vi "mediaIntesecaoBlue.vi"(11 "Array":T4[](array[typedef]) {"robots_blue"."height" format="%+4.3f"; "robots_blue"."pixel_y" format="%+4.3f"; "robots_blue"."pixel_x" format="%+4.3f"; "robots_blue"."orientation" format="%+4.3f"; "robots_blue"."y" format="%+4.3f"; "robots_blue"."confidence" format="%4.3f"; "robots_blue"."x" format="%+4.3f"; "robots_yellow"."height" format="%+4.3f"; "robots_yellow"."pixel_y" format="%+4.3f"; "robots_yellow"."pixel_x" format="%+4.3f"; "robots_yellow"."orientation" format="%+4.3f"; "robots_yellow"."y" format="%+4.3f"; "robots_yellow"."confidence" format="%4.3f"; "robots_yellow"."x" format="%+4.3f"}) -> (3 "Array 2":T1[](array[typedef]) {"height" format="%+4.3f"; "pixel_y" format="%+4.3f"; "pixel_x" format="%+4.3f"; "orientation" format="%+4.3f"; "y" format="%+4.3f"; "confidence" format="%4.3f"; "x" format="%+4.3f"})   [LabVIEW 2018]
uses:
  SSL Detection Frame.ctl
  SSL Detection Robot.ctl
  <vilib>/Analysis/Matrix/Datatypes/RealMatrix.ctl
  SSL Detection Ball.ctl
  <vilib>/Analysis/Matrix/NI_Matrix.lvlib
panel:
  in  "Field Size 2":T3
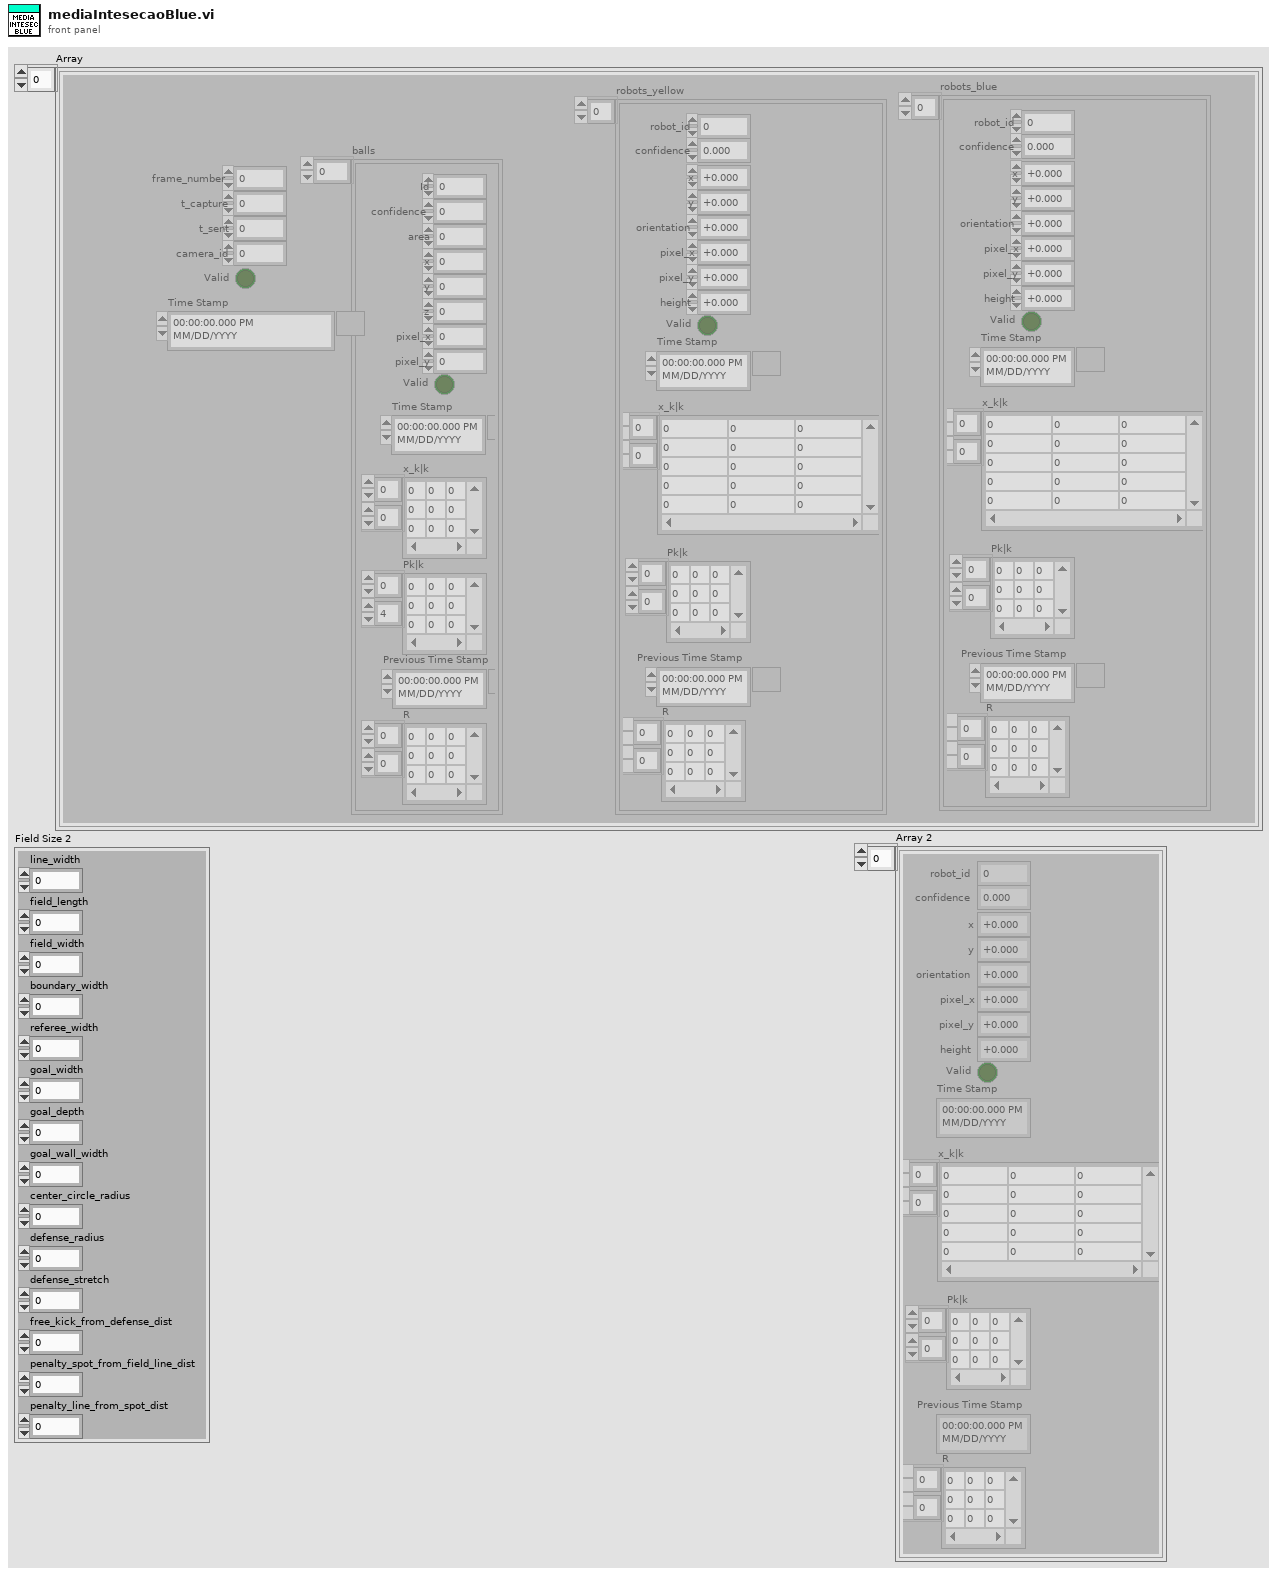
[diagram p1: front panel]
types:
  T1 = typedef "SSL Detection Robot.ctl" = cluster{"x":sgl, "robot_id":u32, "confidence":sgl, "y":sgl, "orientation":sgl, "pixel_x":sgl, "pixel_y":sgl, "height":sgl, "Valid":bool, "Time Stamp":timestamp, "x_k|k":T2, "Pk|k":T2, "Previous Time Stamp":timestamp, "R":T2}
  T2 = typedef "NI_Matrix.lvlib/RealMatrix.ctl" = dbl[][]
  T3 = cluster{"line_width":u32, "field_length":u32, "field_width":u32, "boundary_width":u32, "referee_width":u32, "goal_width":u32, "goal_depth":u32, "goal_wall_width":u32, "center_circle_radius":u32, "defense_radius":u32, "defense_stretch":u32, "free_kick_from_defense_dist":u32, "penalty_spot_from_field_line_dist":u32, "penalty_line_from_spot_dist":u32}
  T4 = typedef "SSL Detection Frame.ctl" = cluster{"frame_number":u32, "t_capture":dbl, "t_sent":dbl, "camera_id":u32, "robots_yellow":T1[], "robots_blue":T1[], "balls":T5[], "Valid":bool, "Time Stamp":timestamp}
  T5 = typedef "SSL Detection Ball.ctl" = cluster{"x":sgl, "area":u32, "confidence":sgl, "y":sgl, "z":sgl, "pixel_x":sgl, "pixel_y":sgl, "Valid":bool, "Time Stamp":timestamp, "x_k|k":T2, "Pk|k":T2, "Id":u32, "Previous Time Stamp":timestamp, "R":T2}
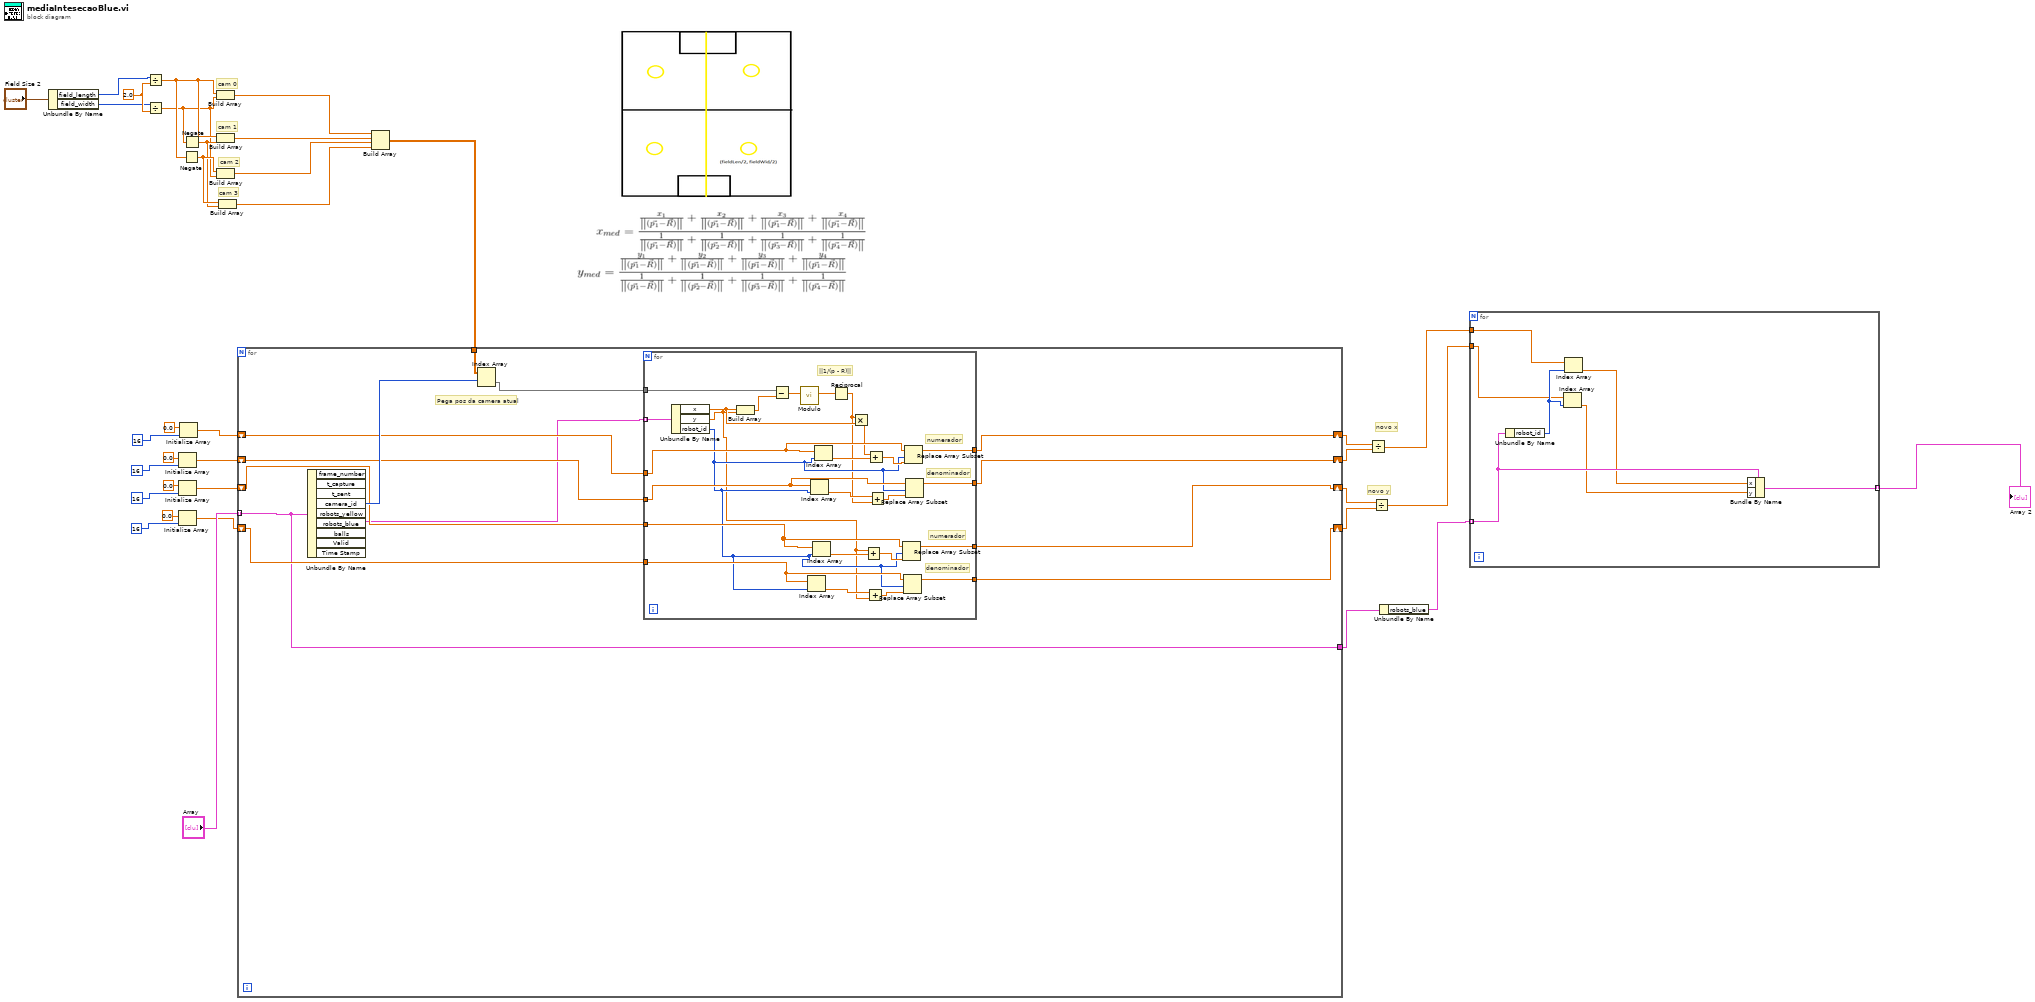
[diagram p0: block diagram]
diagram:
  w33 = 2.0 ("y")
  # "novo y"
  # "novo x"
  # "cam 3"
  # "cam 2"
  # "cam 1"
  # "cam 0"
  n1 = Unbundle By Name("Field Size 2") -> ("field_length"=w32:u32, "field_width"=w31:u32)
  n2 = Divide(x=w32, y=w33) -> (x/y=w29:dbl)
  n3 = Divide(x=w31, y=w33) -> (x/y=w27:dbl)
  n4 = Initialize Array(0.0 ("element"), 16 ("dimension size")) -> (w10:dbl[])
  n5 = Initialize Array(0.0 ("element"), 16 ("dimension size")) -> (w16:dbl[])
  n6 = Initialize Array(0.0 ("element"), 16 ("dimension size")) -> (w11:dbl[])
  n7 = Initialize Array(0.0 ("element"), 16 ("dimension size")) -> (w19:dbl[])
  n8 = Negate(x=w29) -> (-x=w30:dbl)
  n9 = Negate(x=w27) -> (-x=w28:dbl)
  n10 = Build Array(w29, w27) -> (w26:dbl[])
  n11 = Build Array(w29, w28) -> (w25:dbl[])
  n12 = Build Array(w30, w27) -> (w24:dbl[])
  n13 = Build Array(w30, w28) -> (w23:dbl[])
  n14 = Build Array(w26, w25, w24, w23) -> (w22:dbl[][])
  n15 = for {
    tunnel: "Array" -> [w37] mode=indexing
    tunnel: w22 -> [w48]
    shift-right: [w43] -> w9
    shift-left: w19 -> [w45]
    shift-right: [w42] -> w8
    shift-left: w16 -> [w44]
    shift-right: [w39] -> w7
    shift-left: w11 -> [w41]
    shift-right: [w38] -> w6
    shift-left: w10 -> [w40]
    tunnel: [w37] -> w2
    # "Pega pos da camera atual"
    n16 = Unbundle By Name(w37) -> ("camera_id"=w47:u32, "robots_blue"=w36:T1[])  [unwired: 7 out]
    n17 = Index Array(array=w48, index (row)=w47) -> (element=w46:dbl[])  [unwired: 1 in]
    n18 = for {
      tunnel: w36 -> [w74] mode=indexing
      tunnel: w46 -> [w72]
      tunnel: w45 -> [w66]
      tunnel: w44 -> [w62]
      tunnel: [w68] -> w43
      tunnel: [w67] -> w42
      tunnel: w41 -> [w55]
      tunnel: w40 -> [w54]
      tunnel: [w51] -> w39
      tunnel: [w50] -> w38
      # "denominador"
      # "numerador"
      # "denominador"
      # "numerador"
      # "||1/(p - R)||"
      n19 = Unbundle By Name(w74) -> ("x"=w69:sgl, "y"=w49:sgl, "robot_id"=w53:u32)
      n20 = Build Array(w69, w49) -> (w73:sgl[])
      n21 = Subtract(x=w72, y=w73) -> (x-y=w71:dbl[])
      n22 = call "Modulo.vi"("2D vector"=w71) -> ("Modulo"=w70:dbl)  [unwired: 10 in]
      n23 = Index Array(array=w54, index=w53) -> (element=w57:dbl)
      n24 = Index Array(array=w62, index=w53) -> (element=w61:dbl)
      n25 = Index Array(array=w55, index=w53) -> (element=w59:dbl)
      n26 = Index Array(array=w66, index=w53) -> (element=w64:dbl)
      n27 = Reciprocal(x=w70) -> (1/x=w52:dbl)
      n28 = Multiply(x=w52, y=w69) -> (x*y=w65:dbl)
      n29 = Add(x=w49, y=w59) -> (x+y=w58:dbl)
      n30 = Add(x=w57, y=w49) -> (x+y=w56:dbl)
      n31 = Add(x=w65, y=w64) -> (x+y=w63:dbl)
      n32 = Add(x=w61, y=w52) -> (x+y=w60:dbl)
      n33 = Replace Array Subset(array=w55, new element=w58, index=w53) -> (w51:dbl[])
      n34 = Replace Array Subset(array=w54, new element=w56, index=w53) -> (w50:dbl[])
      n35 = Replace Array Subset(array=w66, new element=w63, index=w53) -> (w68:dbl[])
      n36 = Replace Array Subset(array=w62, new element=w60, index=w53) -> (w67:dbl[])
    }
  }
  n37 = Divide(x=w9, y=w8) -> (x/y=w5:dbl[])
  n38 = Divide(x=w7, y=w6) -> (x/y=w4:dbl[])
  n39 = Unbundle By Name(w2) -> ("robots_blue"=w1:T1[])
  n40 = for {
    tunnel: w5 -> [w80]
    tunnel: w4 -> [w78]
    tunnel: w1 -> [w81] mode=indexing
    tunnel: [w75] -> w3 mode=indexing
    n41 = Unbundle By Name(w81) -> ("robot_id"=w79:u32)
    n42 = Index Array(array=w78, index=w79) -> (element=w76:dbl)
    n43 = Index Array(array=w80, index=w79) -> (element=w77:dbl)
    n44 = Bundle By Name(cluster=w81, "x"=w77, "y"=w76) -> (w75:T1)
  }
  "Array 2" <- w3
